vi "poly_time_conversion_s2ms_single.vi"(2 "s":dbl format="%#_13g") -> (7 "ms":i32)   [LabVIEW 2015]
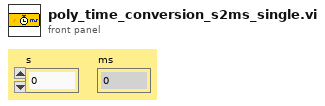
[diagram p1: front panel]
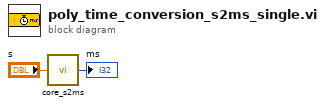
[diagram p0: block diagram]
diagram:
  n1 = call "core_s2ms.vi"("s {DBL}"="s") -> ("ms {I32}"=→"ms":i32)  [unwired: 8 in]
